vi "Create.vi"(8 "error in":errorcluster, 10 "reset":bool, 11 "serial configuration":T1) -> (0 "error out":errorcluster, 3 "session factory out":refnum<class "Session Factory.lvclass">)   [LabVIEW 2021, in "Keysight 34461A DMM Instrument.lvlib" / "Session Factory.lvclass"]
uses:
  Session Factory.lvclass
  Session Factory.lvclass/Session Factory.ctl
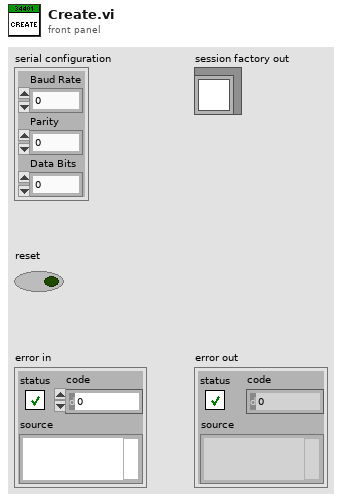
[diagram p1: front panel]
types:
  T1 = cluster{"Baud Rate":u32, "Parity":u16, "Data Bits":u16}
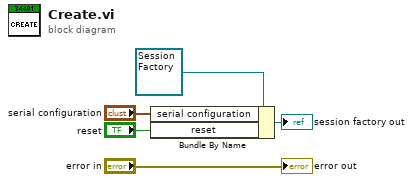
[diagram p0: block diagram]
diagram:
  n1 = Bundle By Name(cluster=refnum<class "Session Factory.lvclass"> refnum ("session factory out"), "serial configuration"="serial configuration", "reset"="reset") -> (→"session factory out":refnum<class "Session Factory.lvclass">)
  "error out" <- "error in"
